vi "Get Wire Prefix.vi"(0 "App Refnum":refnum<vi>, 7 "VI":string, 11 "error in (no error)":errorcluster) -> (4 "Query terms":string[](array[string]), 6 "labVIEW Type":T1, 15 "error out":errorcluster)   [LabVIEW 2018]
doc: "Created by VI-Tech"
uses:
  <vilib>/Utility/Data Type/Type Definitions/Data Type.ctl
  <vilib>/Utility/Data Type/NI_Data Type.lvlib
panel:
  out "Type":enum16{"VI", "Wire"}(ring)
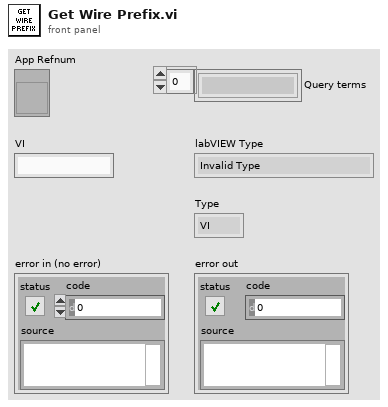
[diagram p1: front panel]
types:
  T1 = typedef "NI_Data Type.lvlib/Data Type.ctl" = enum8{"Invalid Type", "Void", "I8", "I16", "I32", "I64", "U8", "U16", "U32", "U64", "Single Float", "Double Float", "Extended Float", "Single Complex", "Double Complex", "Extended Complex", "Enum U8", "Enum U16", "Enum U32", "Enum U64", "Single Float With Unit", "Double Float With Unit", "Extended Float With Unit", "Single Complex with Unit", "Double Complex with Unit", "Extended Complex with Unit", "Boolean", "String", "Path", "Picture", "Tag", "Array", "Cluster", "Variant", "LV Variant", "Waveform", "Timestamp", "Digital Waveform", "Digital Data", "ExpressData", "Refnum", "External Data", "VI", "Poly VI", "LabVIEW Class Instance", "Fixed Point"}
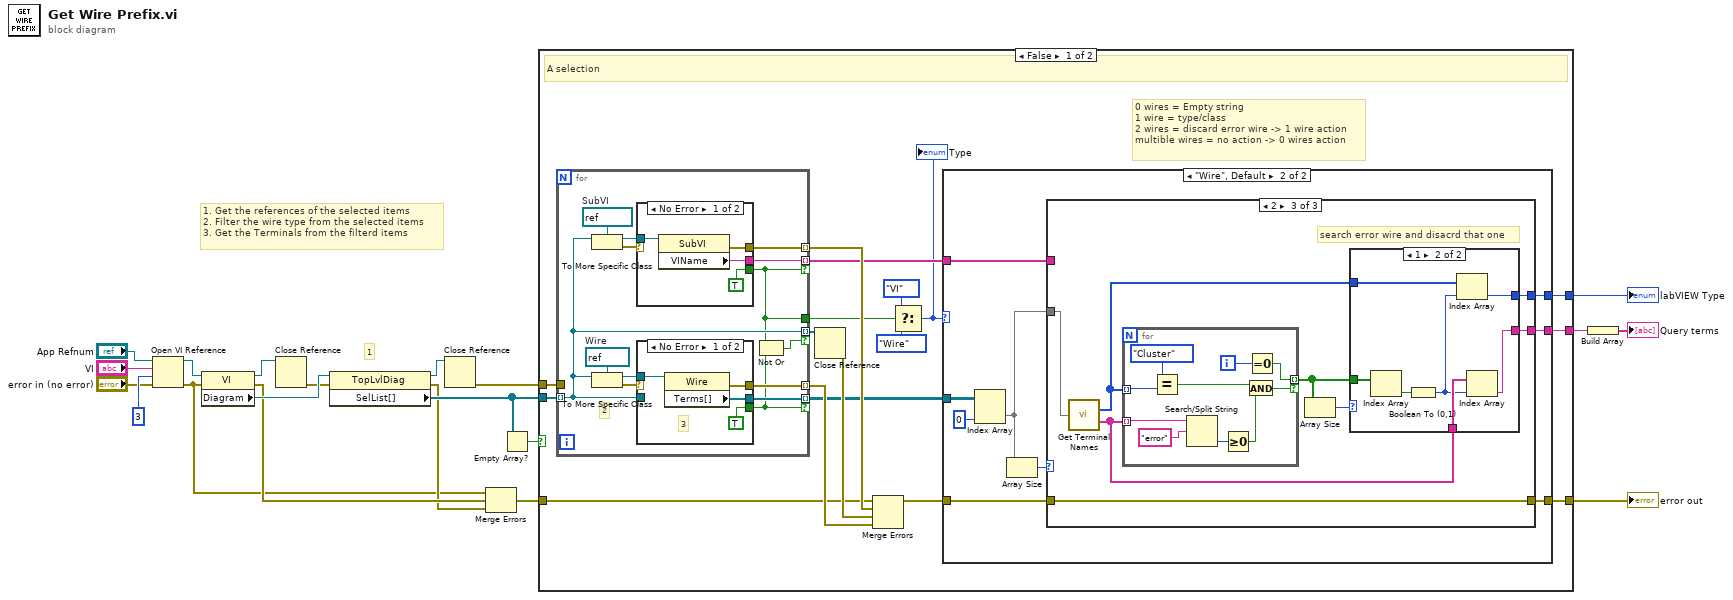
[diagram p0: block diagram]
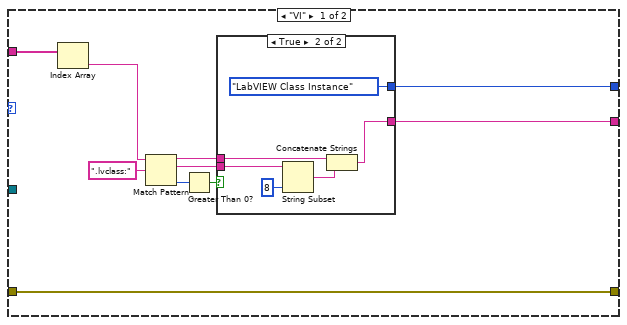
[diagram p2: hidden frame]
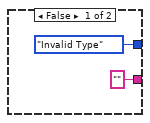
[diagram p3: hidden frame]
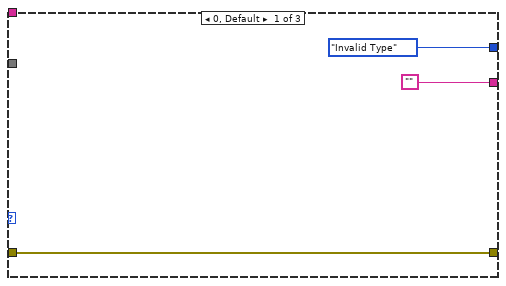
[diagram p4: hidden frame]
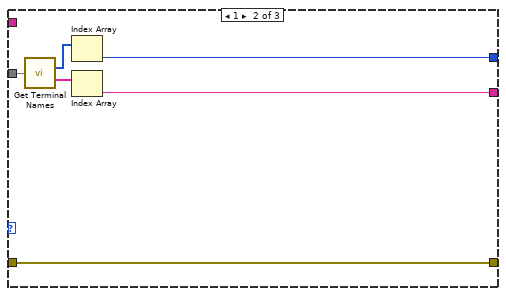
[diagram p5: hidden frame]
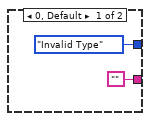
[diagram p6: hidden frame]
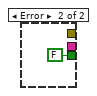
[diagram p7: hidden frame]
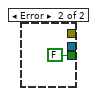
[diagram p8: hidden frame]
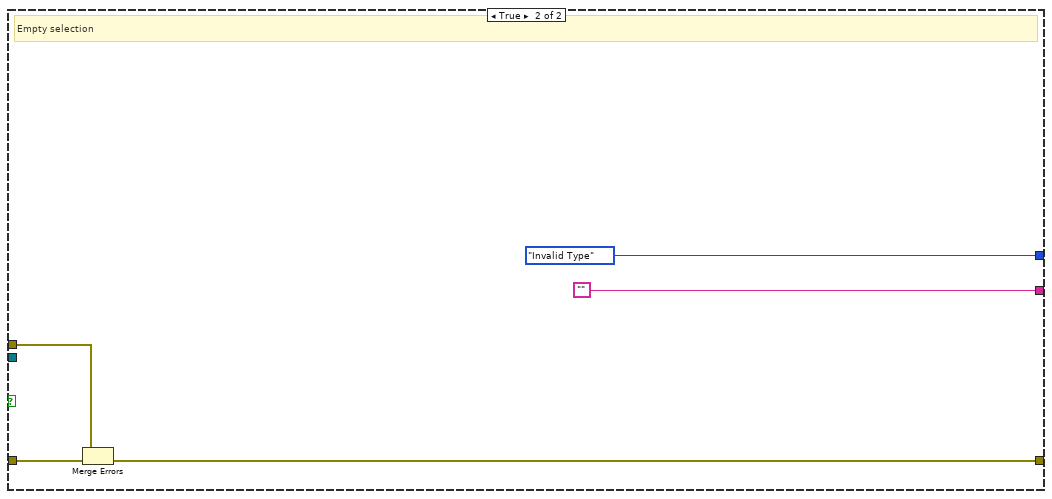
[diagram p9: hidden frame]
diagram:
  # "1"
  # "1. Get the references of the selected items\n2. Filter the wire type from the selected items \n3. Get the Terminals from the filterd items"
  n1 = Open VI Reference(application reference (local)="App Refnum", vi path="VI", options=3, error in (no error)="error in (no error)") -> (vi reference=w17:refnum<vi>, error out=w5:errorcluster)  [unwired: 2 in]
  n2 = property class="VI"(reference=w17, error in=w5) -> (reference out=w16:refnum<vi>, error out=w7:errorcluster, "Diagram"=w19:refnum<vi>)
  n3 = Close Reference(reference=w16) -> (error out=w15:errorcluster)  [unwired: 1 in]
  n4 = property class="TopLvlDiag"(reference=w19, error in=w15) -> (reference out=w20:refnum<vi>, error out=w6:errorcluster, "SelList[]"=w9:refnum<vi>[])
  n5 = Close Reference(reference=w20) -> (error out=w10:errorcluster)  [unwired: 1 in]
  n6 = Merge Errors(w5, w7, w6) -> (w4:errorcluster)
  n7 = Empty Array?(array=w9) -> (empty?=w8:bool)
  n8 = case shown="False" w8 {
    tunnel: w4 -> [w26 w126]
    tunnel: [w37 w125] -> w11
    tunnel: w10 -> [w36 w129]
    tunnel: [w34 "" ("LabVIEW Class File Name")] -> w2
    tunnel: [w33 Data_Type."Invalid Type" ("Type")] -> w3
    tunnel: w9 -> [w32 _]
    frame False {
      # "0 wires = Empty string\n1 wire = type/class\n2 wires = discard error wire -> 1 wire action\nmultible wires = no action -> 0 wires action"
      # "A selection"
      n9 = for {
        tunnel: w32 -> [w108] mode=indexing
        tunnel: w36 -> [_]
        tunnel: [w111] -> w30 mode=indexing
        tunnel: [w108] -> w31 mode=indexing if=w106
        tunnel: [w107] -> w22 mode=indexing if=w101
        tunnel: [w105] -> w29 mode=indexing
        tunnel: [w104] -> w27 mode=indexing if=w102
        tunnel: [w101] -> w23
        w103 = refnum<vi> refnum  # SubVI
        w114 = refnum<vi> refnum  # Wire
        # "2"
        n10 = To More Specific Class(target class=w103, reference=w108) -> (specific class reference=w109:refnum<vi>, error out=w110:errorcluster)  [unwired: 1 in]
        n11 = To More Specific Class(target class=w114, reference=w108) -> (specific class reference=w112:refnum<vi>, error out=w113:errorcluster)  [unwired: 1 in]
        n12 = case shown="No Error" w110 {
          tunnel: w109 -> [w118 _]
          tunnel: [w117 _] -> w107
          tunnel: [w116 _] -> w105
          tunnel: [TRUE FALSE] -> w101
          frame No Error {
            n13 = property class="SubVI"(reference=w118) -> (error out=w116:errorcluster, "VIName"=w117:string)  [unwired: 1 in, 1 out]
          }
          frame Error {
          }
        }
        n14 = case shown="No Error" w113 {
          tunnel: w108 -> [_ _]
          tunnel: w112 -> [w123 _]
          tunnel: [w122 _] -> w104
          tunnel: [w121 _] -> w111
          tunnel: [TRUE FALSE] -> w102
          frame No Error {
            # "3"
            n15 = property class="Wire"(reference=w123) -> (error out=w121:errorcluster, "Terms[]"=w122:refnum<vi>[])  [unwired: 1 in, 1 out]
          }
          frame Error {
          }
        }
        n16 = Not Or(1:w102, 2:w101) -> (0:w106:bool)
      }
      n17 = Close Reference(reference=w31) -> (error out=w28:errorcluster)  [unwired: 1 in]
      n18 = Merge Errors(w26, w29, w28, w30) -> (w35:errorcluster)
      n19 = Select(t=enum16{"VI", "Wire"}."VI", s=w23, f=enum16{"VI", "Wire"}."Wire") -> (s? t:f=w21:enum16{"VI", "Wire"})
      "Type" <- w21
      n20 = case shown="\"Wire\", Default" w21 {
        tunnel: [w47 w64] -> w37
        tunnel: w35 -> [w47 w63]
        tunnel: [w38 w61] -> w34
        tunnel: [w39 w60] -> w33
        tunnel: w27 -> [_ w57]
        tunnel: w22 -> [w46 w56]
        frame "VI" {
          n21 = Index Array(array=w46) -> (element=w45:string)  [unwired: 1 in]
          n22 = Match Pattern(string=w45, regular expression=".lvclass:") -> (before substring=w40:string, match substring=w41:string, offset past match=w43:i32)  [unwired: 1 in, 1 out]
          n23 = Greater Than 0?(x=w43) -> (x > 0?=w42:bool)
          n24 = case shown="True" w42 {
            tunnel: w41 -> [_ w54]
            tunnel: w40 -> [_ w52]
            tunnel: [Data_Type."Invalid Type" ("Type") Data_Type."LabVIEW Class Instance" ("Type")] -> w39
            tunnel: ["" ("LabVIEW Class File Name") w50] -> w38
            frame False {
            }
            frame True {
              n25 = String Subset(string=w54, length (rest)=8 ("length (rest)")) -> (substring=w51:string)  [unwired: 1 in]
              n26 = Concatenate Strings(w52, w51) -> (w50:string)
            }
          }
        }
        frame "Wire", Default {
          n27 = Index Array(array=w57, index (col)=0 ("disabled index (col)")) -> (element=w59:refnum<vi>[])  [unwired: 1 in]
          n28 = Array Size(array=w59) -> (size(s)=w62:i32)
          n29 = case shown="2" w62 {
            tunnel: w59 -> [_ w72 w80]
            tunnel: ["" w70 w77] -> w61
            tunnel: [w66 w73 w81] -> w64
            tunnel: w63 -> [w66 w73 w81]
            tunnel: [Data_Type."Invalid Type" ("Type") w68 w75] -> w60
            tunnel: w56 -> [_ _ _]
            frame 0, Default {
            }
            frame 1 {
              n30 = call "Get Terminal Names.vi"("Input Terms[]"=w72) -> ("Type"=w69:T1[], "Name"=w71:string[])  [unwired: 13 in]
              n31 = Index Array(array=w69) -> (element=w68:T1)  [unwired: 1 in]
              n32 = Index Array(array=w71) -> (element=w70:string)  [unwired: 1 in]
            }
            frame 2 {
              # "search error wire and disacrd that one"
              n33 = call "Get Terminal Names.vi"("Input Terms[]"=w80) -> ("Type"=w74:T1[], "Name"=w76:string[])  [unwired: 13 in]
              n34 = for {
                tunnel: w74 -> [w91] mode=indexing
                tunnel: w76 -> [w88] mode=indexing
                tunnel: [w82] -> w78 mode=indexing if=w84
                i -> [w83]
                n35 = Equal?(x=Data_Type."Cluster" ("Type"), y=w91) -> (x = y?=w85:bool)
                n36 = Search/Split String(string=w88, search string/char (-)="error") -> (offset of match=w87:i32)  [unwired: 1 in, 2 out]
                n37 = Greater Or Equal To 0?(x=w87) -> (x >= 0?=w86:bool)
                n38 = And(x=w85, y=w86) -> (x .and. y?=w84:bool)
                n39 = Equal To 0?(x=w83) -> (x = 0?=w82:bool)
              }
              n40 = Array Size(array=w78) -> (size(s)=w79:i32)
              n41 = case shown="1" w79 {
                tunnel: w78 -> [_ w98]
                tunnel: ["" w100] -> w77
                tunnel: w76 -> [_ w99]
                tunnel: [Data_Type."Invalid Type" ("Type") w96] -> w75
                tunnel: w74 -> [_ w94]
                frame 0, Default {
                }
                frame 1 {
                  n42 = Index Array(array=w98) -> (element=w97:bool)  [unwired: 1 in]
                  n43 = Boolean To (0,1)(Boolean=w97) -> (0, 1=w95:i16)
                  n44 = Index Array(array=w94, index=w95) -> (element=w96:T1)
                  n45 = Index Array(array=w99, index=w95) -> (element=w100:string)
                }
              }
            }
          }
        }
      }
    }
    frame True {
      # "Empty selection"
      n46 = Merge Errors(w129, w126) -> (w125:errorcluster)
    }
  }
  "error out" <- w11
  "labVIEW Type" <- w3
  n47 = Build Array(w2) -> (→"Query terms":string[])
